vi "ActBalance.vi"(10 "MaxSpeed (ft/s)":dbl) -> (0 "RightSpeedDemand":dbl, 1 "LeftSpeedDemand":dbl, 3 "Done":bool)   [LabVIEW 2020]
doc: "Drive the robot straight in arcade drive\nList of things to tune:\n-MaxSpeed\n-ErrorThresh\n-ErrorDead\n-MinOutput\n-MaxOutput\n-Count\n\nInputs:\n--Dist -- Double -- in feet, the distance you want to go when you push the joystick (Get this value from human input)\n-- MaxSpeed -- Double -- in ft/s, the MaxSpeed the robot can go (NEEDS TO BE TUNED)\n-- First Time - Bool -- is this the first time the distance is changing? \n\nOutputs:\n-- Done -- Bool -- has the robot reached its target distance\n-- Unfilt. L Target -- Bool -- unfilteredOnTarget for Left, for debugging purposes\n-- Unfilt. R Target -- Bool -- unfilteredOnTarget for Right, for debugging purposes"
uses:
  <vilib>/Rock Robotics/WPI/ThirdParty/JAS_Junk/TrajLib/LinearFilter_ResetToValue.vi
  <vilib>/Rock Robotics/WPI/ThirdParty/JAS_Junk/TrajLib/LinearFilter_Calculate.vi
  <vilib>/Rock Robotics/Network Tables/NT Write Number.vi
  <vilib>/Rock Robotics/WPI/ThirdParty/JAS_Junk/TrajLib/LinearFilter_MovingAverage.vi
  <vilib>/Rock Robotics/WPI/ThirdParty/JAS_Junk/TrajLib/LinearFilter_LowPassBW1.vi
  <vilib>/Rock Robotics/WPI/ThirdParty/JAS_Junk/TrajLib/LinearFilter_LowPassBW2.vi
  <vilib>/Rock Robotics/WPI/ThirdParty/JAS_Junk/TrajLib/LinearFilter_HighPassBW1.vi
  <vilib>/Rock Robotics/WPI/ThirdParty/JAS_Junk/TrajLib/LinearFilter_HighPassBW2.vi
  <vilib>/Rock Robotics/WPI/ThirdParty/JAS_Junk/TrajLib/Trajectory_Library.lvlib
  <vilib>/Rock Robotics/Network Tables/NT Write Boolean.vi
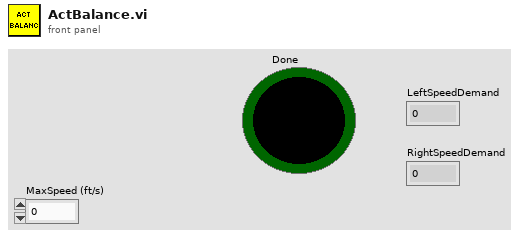
[diagram p1: front panel]
types:
  T1 = enum16{"Moving Average", "Low Pass 1st Order Butterworth", "Low Pass 2nd Order Butterworth", "High Pass 1st Order Butterworth", "High Pass 2nd Order Butterworth"}
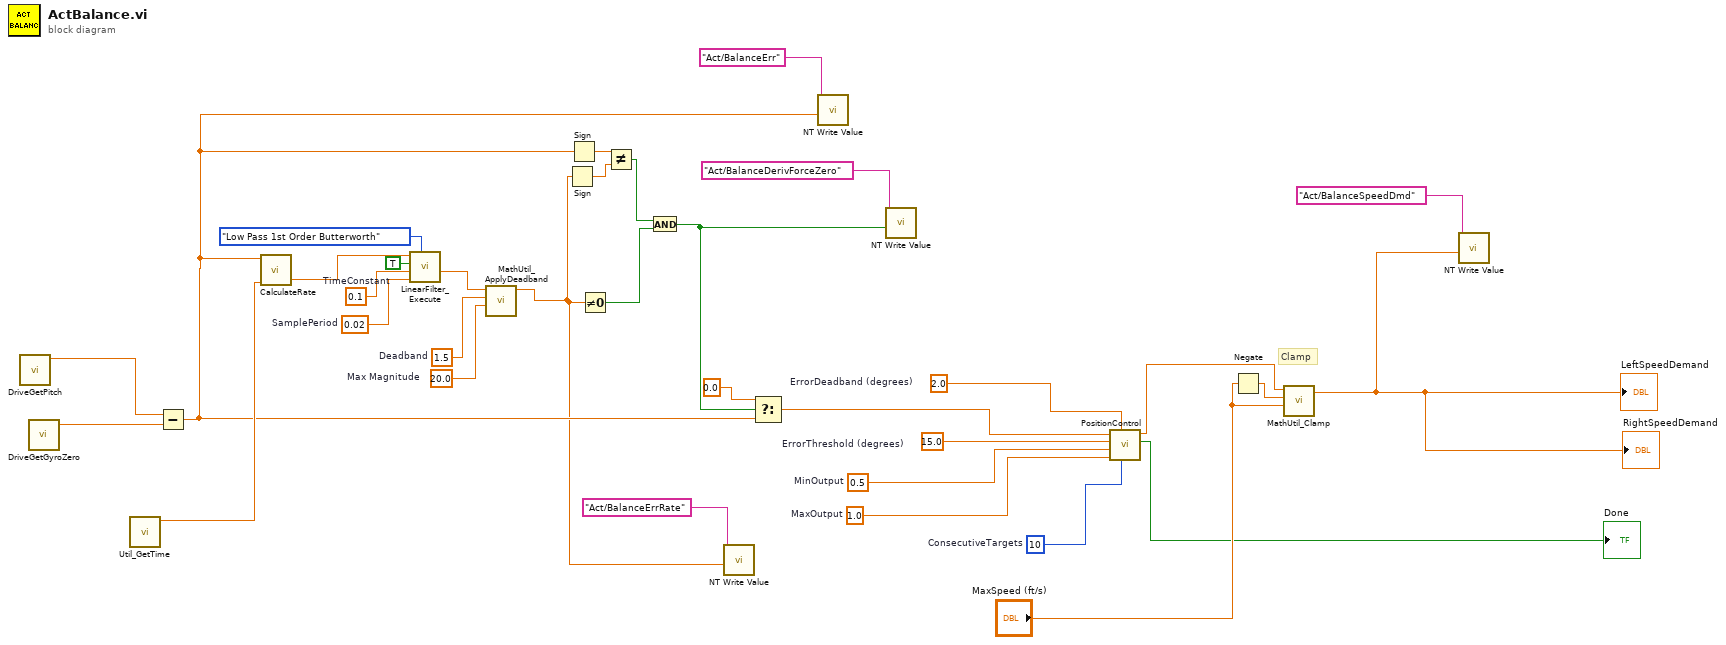
[diagram p0: block diagram]
diagram:
  w15 = 0.02  # SamplePeriod
  w14 = 0.1  # TimeConstant
  w16 = 20.0  # Max Magnitude
  w17 = 1.5  # Deadband
  w28 = 1.0  # MaxOutput
  w29 = 0.5  # MinOutput
  w26 = 10  # ConsecutiveTargets
  w33 = 2.0  # ErrorDeadband (degrees)
  w34 = 15.0  # ErrorThreshold (degrees)
  # "Clamp"
  n1 = call "DriveGetPitch.vi"() -> ("Pitch"=w24:dbl)  [unwired: 11 in]
  n2 = call "DriveGetGyroZero.vi"() -> ("GyroZero"=w25:dbl)  [unwired: 11 in]
  n3 = call <vilib>:"Util_GetTime.vi"() -> ("FPGA_Time_Seconds"=w18:dbl)  [unwired: 10 in, 1 out]
  n4 = Subtract(x=w24, y=w25) -> (x-y=w8:dbl)
  n5 = call "CalculateRate.vi"("Time (s)"=w18, "Distance (units)"=w8) -> ("Rate (units/s)"=w7:dbl)  [unwired: 9 in]
  n6 = call <vilib>:"LinearFilter_Execute.vi"("Filter Type"=T1."Low Pass 1st Order Butterworth", "SamplePeriod"=w15, "TimeConstant"=w14, "Enable"=TRUE, "Input"=w7) -> ("Output"=w6:dbl)  [unwired: 5 in, 1 out]
  n7 = call <vilib>:"MathUtil_ApplyDeadband.vi"("Max Magnitude"=w16, "Deadband"=w17, "Value"=w6) -> ("Result"=w5:dbl)  [unwired: 8 in]
  n8 = Sign(1:w5) -> (0:w21:dbl)
  n9 = Sign(1:w8) -> (0:w22:dbl)
  n10 = Not Equal To 0?(x=w5) -> (x != 0?=w11:bool)
  n11 = Not Equal?(x=w22, y=w21) -> (x != y?=w20:bool)
  n12 = And(x=w20, y=w11) -> (x .and. y?=w3:bool)
  n13 = call-poly <vilib>:"NT Write Value.vi"("value"=w5, "name"="Act/BalanceErrRate") -> ()  [unwired: 9 in, 1 out]
  n14 = Select(t=0.0, s=w3, f=w8) -> (s? t:f=w19:dbl)
  n15 = call-poly <vilib>:"NT Write Value.vi"("value"=w8, "name"="Act/BalanceErr") -> ()  [unwired: 9 in, 1 out]
  n16 = call-poly <vilib>:"NT Write Value.vi"("value"=w3, "name"="Act/BalanceDerivForceZero") -> ()  [unwired: 9 in, 1 out]
  n17 = call "PositionControl.vi"("ConsecutiveTargets"=w26, "ErrorDeadband"=w33, "MaxOutput"=w28, "MinOutput"=w29, "ErrorThreshold"=w34, "Error"=w19) -> ("OnTarget"=→"Done":bool, "OutputValue"=w32:dbl)  [unwired: 3 in, 1 out]
  n18 = Negate(x="MaxSpeed (ft/s)") -> (-x=w31:dbl)
  n19 = call <vilib>:"MathUtil_Clamp.vi"("High Limit"="MaxSpeed (ft/s)", "Low Limit"=w31, "Value"=w32) -> ("Result"=w1:dbl)  [unwired: 8 in]
  "LeftSpeedDemand" <- w1
  "RightSpeedDemand" <- w1
  n20 = call-poly <vilib>:"NT Write Value.vi"("value"=w1, "name"="Act/BalanceSpeedDmd") -> ()  [unwired: 9 in, 1 out]
